vi "Echo_Global_Data.vi"() -> ()   [LabVIEW 2012]
doc: "This global VI can contain as many global variables as you need. Place a control on the panel, give it a good name. To read or write to it from a VI, drag the icon to the diagram of that VI. You can also drag from the project. Click on the node to change which global you access. You shouldn't have multiple locations writing to a global or it will cause a race-condition."
panel:
  in  "Autonomous Mode":path[](array[path])
  in  "Echo Combined Data":dbl[][][](array[numeric])
  in  "Echo Recorded Data 10":dbl
  in  "Echo Recorded Data 09":dbl
  in  "Echo Recorded Data 08":dbl
  in  "Echo Recorded Data 07":dbl
  in  "Echo Recorded Data 06":dbl
  in  "Echo Recorded Data 05":dbl
  in  "Echo Recorded Data 04":dbl
  in  "Echo Recorded Data 03":dbl
  in  "Echo Recorded Data 02":dbl
  in  "Echo Recorded Data 01":dbl
  # "This 3D array is read from and \nindexed to create the outputs in\nEcho Autonomous Independent.\n\nIt is written to by Echo Begin and\nEcho Periodic Tasks.\n\nIt contains the data from several\n2D spreadsheets, each \nrepresenting a single routine\n\nIts dimensions are N x 250 x 11,\nN is the number of routines to \nbe run."
  # "These Global Variables represent the current values of \nthe data that will be written to in Teleop or Periodic Tasks\nand will be saved to a spreadsheet representing a routine."
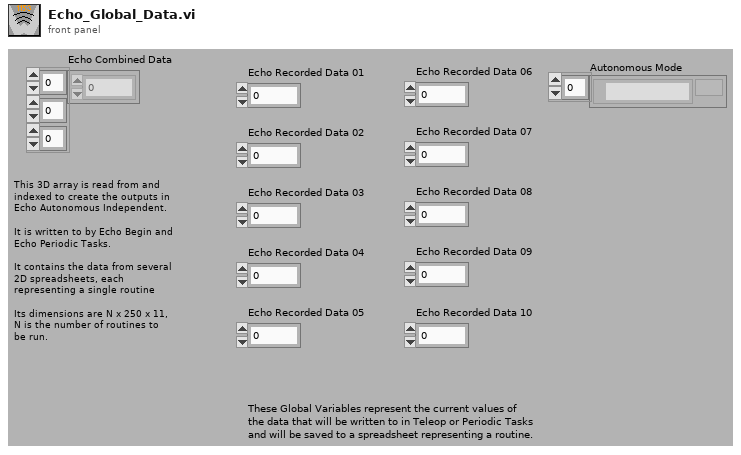
[diagram p1: front panel]
diagram:
